vi "Save config files backup.vi"(8 "error in (no error)":errorcluster) -> (0 "error out":errorcluster)   [LabVIEW 2020]
uses:
  Typedefs/HW config states enum.ctl
  Typedefs/Save-Load enum.ctl
  Global Variables/General Globals.vi
panel:
  out "x-y":u32
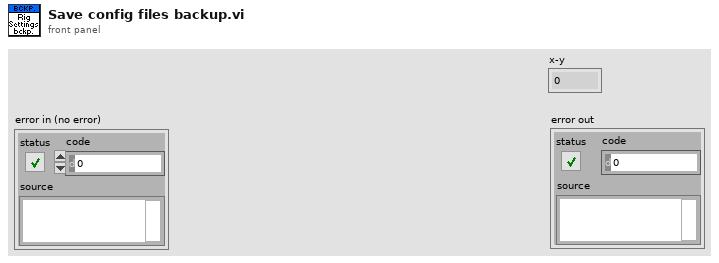
[diagram p1: front panel]
types:
  T1 = typedef "Save-Load enum.ctl" = enum16{"Save to file", "Load from file", "Compare from file", "Save Backup"}
  T2 = enum16{"Initialise", "Load from file", "Save to file", "Read", "Write"}
  T3 = typedef "HW config states enum.ctl" = enum16{"Load from file", "Save to file", "Save backup", "Write all", "Read all", "Write XY stage settings", "Write DAQ FPGA settings", "Write Control FPGA settings", "Write Phys Channels", "Write System Config", "Write HW Config", "Save System Config", "Save HW Config", "Clear", "Compare from file"}
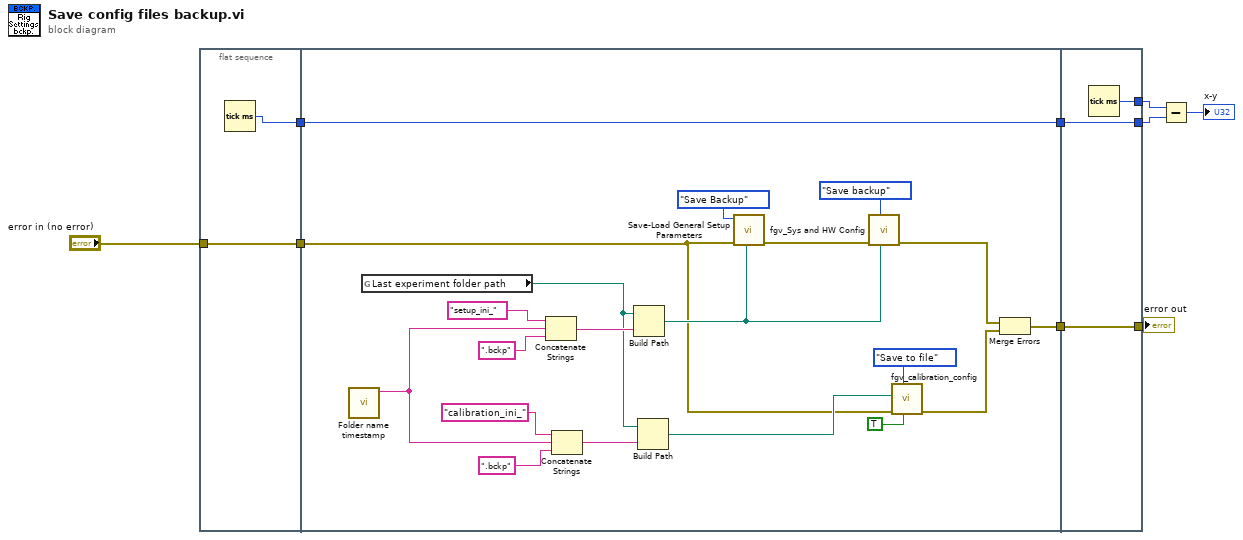
[diagram p0: block diagram]
diagram:
  n1 = flat-sequence {
    tunnel: "error in (no error)" -> [w11]
    tunnel: [w11] -> w6
    tunnel: [w10] -> w4
    tunnel: [w14] -> w7
    tunnel: w6 -> [w17]
    tunnel: [w12] -> w5
    tunnel: w4 -> [w12]
    tunnel: [w34] -> w8
    tunnel: w7 -> [w34]
    tunnel: [w33] -> w3
    tunnel: [w32] -> w2
    tunnel: w5 -> [w32]
    frame #0 {
      n2 = Tick Count (ms)() -> (millisecond timer value=w10:u32)
    }
    frame #1 {
      n3 = call "Folder name timestamp.vi"() -> ("date/time string"=w23:string)  [unwired: 11 in]
      n4 = global read "General Globals.vi" "Last experiment folder path"() -> (w13:path)
      n5 = Concatenate Strings("setup_ini_" ("name or relative path"), w23, ".bckp" ("string")) -> (w30:string)
      n6 = Concatenate Strings("calibration_ini_" ("string"), w23, ".bckp" ("string")) -> (w24:string)
      n7 = Build Path(base path=w13, name or relative path=w30) -> (appended path=w19:path)
      n8 = Build Path(base path=w13, name or relative path=w24) -> (appended path=w21:path)
      n9 = call "Save-Load General Setup Parameters.vi"("backup file path"=w19, "error in"=w17, "Function"=Save-Load_enum."Save Backup") -> ("error out"=w18:errorcluster)  [unwired: 8 in]
      n10 = call "fgv_Sys and HW Config.vi"("backup file path"=w19, "Function"=HW_config_states_enum."Save backup", "error in (no error)"=w18) -> ("error out"=w16:errorcluster)  [unwired: 6 in, 2 out]
      n11 = call "fgv_calibration_config.vi"("Non default file path?"=TRUE, "Cal config ops"=T2."Save to file", "error in (no error)"=w17, "config file path"=w21) -> ("error out"=w15:errorcluster)  [unwired: 5 in, 2 out]
      n12 = Merge Errors(w16, w15) -> (w14:errorcluster)
    }
    frame #2 {
      n13 = Tick Count (ms)() -> (millisecond timer value=w33:u32)
    }
  }
  n14 = Subtract(x=w3, y=w2) -> (x-y=→"x-y":u32)
  "error out" <- w8
